vi "TTA_EXA_SetEXA4TxOutputTest.vi"(0 "VISA resource In":refnum<visa-resource-name>, 1 "Reference Level (dBm)":dbl, 5 "Frequency (MHz)":dbl, 7 "Span (kHz)":dbl, 9 "RBW (Hz)":dbl, 11 "error in":errorcluster) -> (4 "VISA resource Out":refnum<visa-resource-name>, 15 "error out":errorcluster)   [LabVIEW 2016]
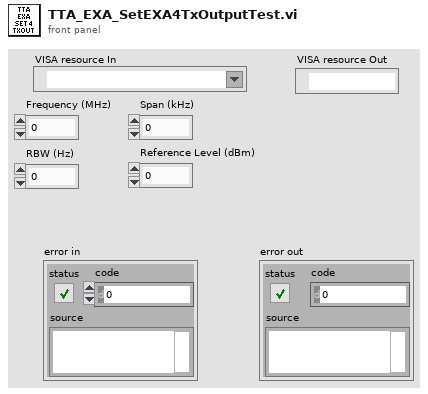
[diagram p1: front panel]
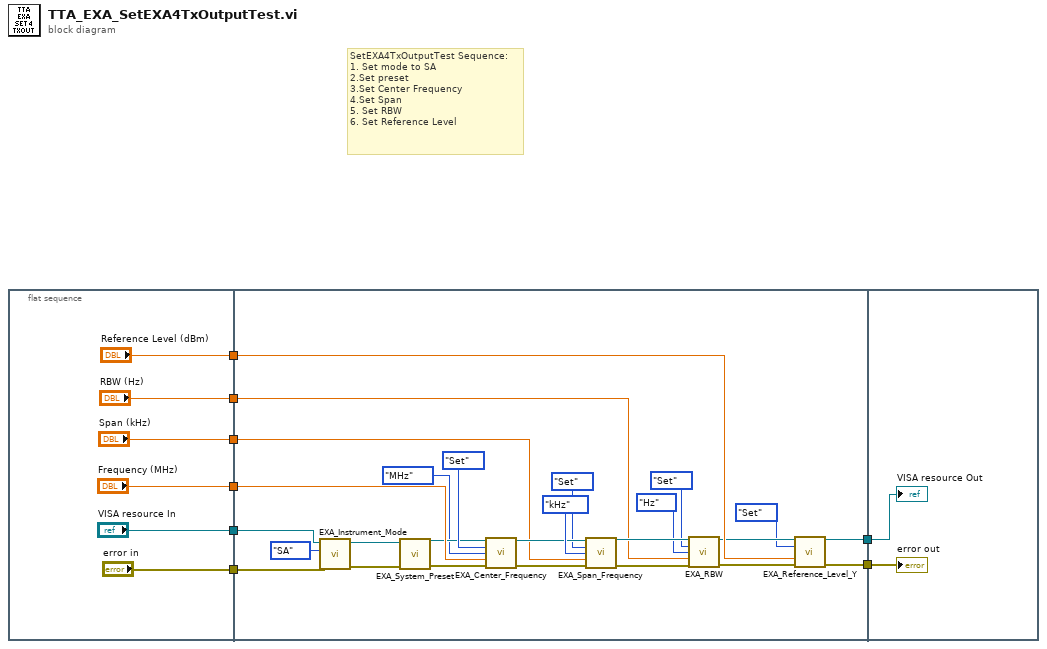
[diagram p0: block diagram]
diagram:
  # "SetEXA4TxOutputTest Sequence:\n1. Set mode to SA\n2.Set preset\n3.Set Center Frequency\n4.Set Span\n5. Set RBW\n6. Set Reference Level"
  n1 = flat-sequence {
    tunnel: ["error in"] -> w8
    tunnel: ["VISA resource In"] -> w7
    tunnel: ["Frequency (MHz)"] -> w6
    tunnel: ["Span (kHz)"] -> w5
    tunnel: ["RBW (Hz)"] -> w4
    tunnel: ["Reference Level (dBm)"] -> w3
    tunnel: w8 -> [w37]
    tunnel: w7 -> [w36]
    tunnel: w6 -> [w30]
    tunnel: w5 -> [w26]
    tunnel: w4 -> [w21]
    tunnel: w3 -> [w19]
    tunnel: [w16] -> w2
    tunnel: [w15] -> w1
    tunnel: w2 -> [w42]
    tunnel: w1 -> [w41]
    frame #0 {
    }
    frame #1 {
      n2 = call "EXA_Instrument_Mode.vi"("error in"=w37, "Mode"=enum16{"SA", "LTE"}."SA", "VISA resource name"=w36) -> ("error out"=w40:errorcluster, "VISA resource name"=w39:refnum<visa-resource-name>)  [unwired: 7 in]
      n3 = call "EXA_System_Preset.vi"("error in"=w40, "VISA resource name"=w39) -> ("error out"=w35:errorcluster, "VISA resource name"=w28:refnum<visa-resource-name>)  [unwired: 8 in]
      n4 = call "EXA_Center_Frequency.vi"("VISA resource name"=w28, "Mode"=enum16{"Set", "Get"}."Set", "Units"=enum16{"Hz", "kHz", "MHz", "GHz"}."MHz", "Frequency"=w30, "error in"=w35) -> ("VISA resource name"=w32:refnum<visa-resource-name>, "error out"=w33:errorcluster)  [unwired: 8 in, 1 out]
      n5 = call "EXA_Span_Frequency.vi"("VISA resource name"=w32, "Mode"=enum16{"Set", "Get"}."Set", "Units"=enum16{"Hz", "kHz", "MHz", "GHz"}."kHz", "Span"=w26, "error in"=w33) -> ("VISA resource name"=w24:refnum<visa-resource-name>, "error out"=w25:errorcluster)  [unwired: 8 in, 1 out]
      n6 = call "EXA_RBW.vi"("VISA resource name"=w24, "Mode"=enum16{"Set", "Get"}."Set", "Units"=enum16{"Hz", "kHz", "MHz", "GHz"}."Hz", "RBW"=w21, "error in"=w25) -> ("VISA resource name"=w18:refnum<visa-resource-name>, "error out"=w20:errorcluster)  [unwired: 8 in, 1 out]
      n7 = call "EXA_Reference_Level_Y.vi"("VISA resource name"=w18, "Mode"=enum16{"Set", "Get"}."Set", "Reference Level (dBm)"=w19, "error in"=w20) -> ("VISA resource name"=w16:refnum<visa-resource-name>, "error out"=w15:errorcluster)  [unwired: 9 in, 1 out]
    }
    frame #2 {
      "VISA resource Out" <- w42
      "error out" <- w41
    }
  }
